vi "Main Read Data From VeriStand.vi"(8 "error in (no error)":errorcluster, 11 "J1939 Main Configuration":T1={"Parameters"={"J1939 XNET Settings"={"XNET Database"="", "XNET Cluster"="", "CAN Port"="", "Baud rate [Bd]"=0, "Termination"=0, "Incoming Rate"=0, "Outcoming Rate"=1, "Write Decimation"=1}, "Incoming Single Point Configuraiton"={"Incoming Single Point Frame"={"ID"=[], "Conversion"=[], "Channel Array Positions"=[], "Frame Length"=[]}, "Channel Pairs"={"Chan Refs"=[], "Previous Chan Values"=[]}, "Read FIFO"=refnum}, "Outgoing Cyclic Configuraiton"={"Outgoing Cyclic Frame"={"ID"=[], "Conversion"=[], "Channel Array Positions"=[], "Frame Length"=[], "Transmit Propreties"=[]}, "Channel Pairs"={"Block Data Refs"=[], "Previous Chan Values"=[]}, "Write FIFO"=refnum}, "J1939 Monitor Settings"={"J1939 Network Address"=0, "Name"=0}, "Simulated Addresses"=[], "Simulated Addresses LUT"=variant}, "Name"="", "J1939 Cluster"={"Processed Incoming"=refnum, "Current Device Address"=0, "Processed Outgoing"=refnum, "Process Outgoing"=refnum, "Name"=0}, "References"={"BAM Buffer"=refnum, "CM Buffer"=refnum, "CM Gen"=refnum, "BAM Gen"=refnum, "Address Claims"=refnum, "RQST"=refnum}, "StopRef"=refnum, "Frame In"="", "Frame Out"="", "Incoming Timeout"=0, "Outgoing Timeout"=0, "Listener ID"=refnum, "Parent VI Ref"=refnum, "Data Ref"=refnum, "Scale Ref"=refnum, "Incoming Direct Access"={"Offset"=0, "Length"=0}, "Outgoing Direct Access"={"Offset"=0, "Length"=0}, "vi reference"=refnum, "Name and Address"="", "Simulated Addresses"=[], "Simulated Addresses LUT"=variant} {"Simulated Addresses"."Simulated Addresses"."J1939 XNET Settings"."Name" format="%.0x"; "Simulated Addresses"."Simulated Addresses"."DM1 Data"."Data Reference" format="%.0x"; "Simulated Addresses"."Simulated Addresses"."DM1 Enable?"."Data Reference" format="%.0x"; "Simulated Addresses"."Simulated Addresses"."DM2 Data"."Data Reference" format="%.0x"; "Simulated Addresses"."Simulated Addresses"."DM2 Enable?"."Data Reference" format="%.0x"; "Parameters"."Simulated Addresses"."Simulated Addresses"."J1939 XNET Settings"."Name" format="%.0x"; "Parameters"."J1939 Monitor Settings"."Name" format="%.0x"; "Parameters"."Outgoing Cyclic Configuraiton"."Channel Pairs"."Block Data Refs"."Data Reference" format="%.0x"; "Parameters"."Outgoing Cyclic Configuraiton"."Outgoing Cyclic Frame"."Transmit Propreties"."Transmit Time" format="%#_p"; "Parameters"."J1939 XNET Settings"."Termination" items=["Off", "On"]; "Parameters"."Incoming Single Point Configuraiton"."Channel Pairs"."Chan Refs" format="%.0x"}) -> (0 "error out":errorcluster)   [LabVIEW 2013, in "J1939 Addon Engine.lvlib"]
uses:
  J1939 Addon Engine.lvlib
  Types/Configuration Cluster.ctl
  Types/Process Parameters.ctl
  Shared/Types/XNET Settings.ctl
  Types/Incoming Single Point Configuration.ctl
  Types/Incoming Single Point Frame Pairs.ctl
  Types/Incoming Single Point Channel Pairs.ctl
  <vilib>/NI Veristand/Custom Device API/Data Reference.ctl
  Types/Outgoing Cyclic Configuration.ctl
  Types/Outgoing Cyclic Frame Pairs.ctl
  Shared/Types/XNET Frame Event Properties.ctl
  Types/Outgoing Cyclic Channel Pairs.ctl
  <vilib>/NI Veristand/Custom Device API/Block Data Reference.ctl
  Shared/Types/Monitor Settings.ctl
  Types/Simulated Settings.ctl
  Shared/Types/Compiled Simulated Settings.ctl
  Types/DTC FIFOs.ctl
  Shared/J1939 Multi Packet Frame/Types/Setup Information Cluster.ctl
  <vilib>/xnet/xnet.llb/XNET Frame CAN.ctl
  <vilib>/xnet/xnet.llb/XNET Frame Type CAN.ctl
  Shared/J1939 Utilities/Types/CAN Outgoing Message Cluster.ctl
  Shared/J1939 Multi Packet Frame/Types/TP List References.ctl
  Shared/J1939 Multi Packet Frame/Types/BAM Buffer Connections List_Ref.ctl
  Shared/J1939 Multi Packet Frame/Types/Connection Mode Generation Connection Ref.ctl
  Shared/J1939 Multi Packet Frame/Types/BAM Generation Connections List_Ref.ctl
  Shared/J1939 Multi Packet Frame/Types/Address Table Reference.ctl
  Shared/J1939 Multi Packet Frame/Types/RQST Lookup Table Reference.ctl
  Stop FG/Stop Global Ref.ctl
  Diagnostics Addon/Source/Engine/SubVIs/Datatable Lookup DVR.ctl
  Shared/J1939 Multi Packet Frame/Types/RQST Comm Lookup Table_Ref.ctl
  Stop FG/Stop Global Commands.ctl
  Conversion Lookup Table Get Conversion Parameter.vi
  Data Lookup Table.vi
  Conversion Lookup Table.vi
  <vilib>/xnet/xnet.llb/XNET Convert.vi
  <vilib>/xnet/xnet.llb/XNET Convert (Signal to Frame Raw).vi
  Stop FG/Stop FG.lvlib
  Error Handling API/Error Handling API.lvlib
  Shared/J1939 Utilities/J1939 Utilities.lvlib
  <vilib>/NI Veristand/Custom Device API/Custom Device API.lvlib
  Shared/J1939 Addon Shared.lvlib
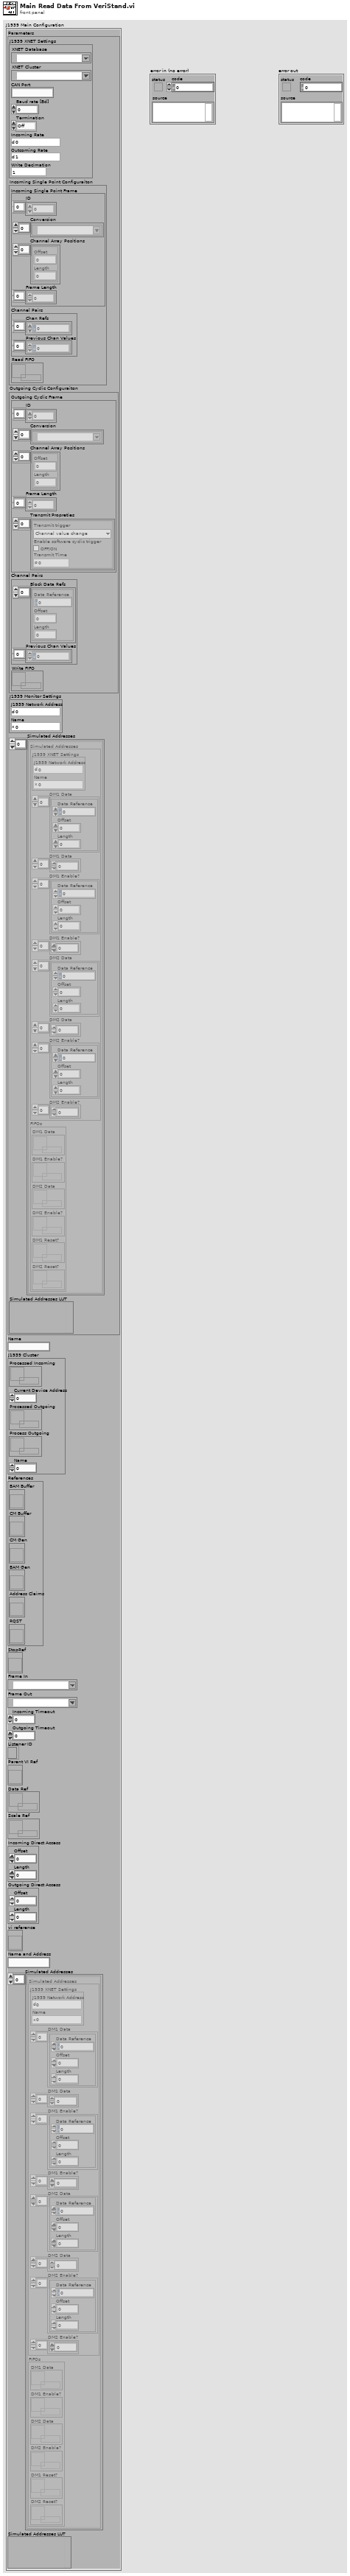
[diagram p1: front panel]
types:
  T1 = typedef "J1939 Addon Engine.lvlib/Configuration Cluster.ctl" = cluster{"Parameters":T2, "Name":string, "J1939 Cluster":T17, "References":T18, "StopRef":T24, "Frame In":refnum<k21>, "Frame Out":refnum<k21>, "Incoming Timeout":u32, "Outgoing Timeout":u32, "Listener ID":refnum<k5>, "Parent VI Ref":refnum<vi>, "Data Ref":refnum<data-value>, "Scale Ref":refnum<data-value>, "Incoming Direct Access":cluster{"Offset":u32, "Length":u32}, "Outgoing Direct Access":cluster{"Offset":u32, "Length":u32}, "vi reference":T25, "Name and Address":string, "Simulated Addresses":T14[], "Simulated Addresses LUT":variant}
  T2 = typedef "J1939 Addon Engine.lvlib/Process Parameters.ctl" = cluster{"J1939 XNET Settings":T3, "Incoming Single Point Configuraiton":T4, "Outgoing Cyclic Configuraiton":T8, "J1939 Monitor Settings":T13, "Simulated Addresses":T14[], "Simulated Addresses LUT":variant}
  T3 = typedef "J1939 Addon Shared.lvlib/XNET Settings.ctl" = cluster{"XNET Database":refnum<k21>, "XNET Cluster":refnum<k21>, "CAN Port":string, "Baud rate [Bd]":u32, "Termination":u32, "Incoming Rate":u32, "Outcoming Rate":u32, "Write Decimation":u32}
  T4 = typedef "J1939 Addon Engine.lvlib/Incoming Single Point Configuration.ctl" = cluster{"Incoming Single Point Frame":T5, "Channel Pairs":T6, "Read FIFO":refnum<k33>}
  T5 = typedef "J1939 Addon Engine.lvlib/Incoming Single Point Frame Pairs.ctl" = cluster{"ID":u32[], "Conversion":refnum<k21>[], "Channel Array Positions":cluster{"Offset":u32, "Length":u32}[], "Frame Length":u32[]}
  T6 = typedef "J1939 Addon Engine.lvlib/Incoming Single Point Channel Pairs.ctl" = cluster{"Chan Refs":T7[], "Previous Chan Values":dbl[]}
  T7 = typedef "Custom Device API.lvlib/Data Reference.ctl" = i32
  T8 = typedef "J1939 Addon Engine.lvlib/Outgoing Cyclic Configuration.ctl" = cluster{"Outgoing Cyclic Frame":T9, "Channel Pairs":T11, "Write FIFO":refnum<k33>}
  T9 = typedef "J1939 Addon Engine.lvlib/Outgoing Cyclic Frame Pairs.ctl" = cluster{"ID":u32[], "Conversion":refnum<k21>[], "Channel Array Positions":cluster{"Offset":u32, "Length":u32}[], "Frame Length":u32[], "Transmit Propreties":T10[]}
  T10 = typedef "J1939 Addon Shared.lvlib/XNET Frame Event Properties.ctl" = cluster{"Transmit trigger":enum16{"Channel value change"}, "Enable software cyclic trigger":bool, "Transmit Time":dbl}
  T11 = typedef "J1939 Addon Engine.lvlib/Outgoing Cyclic Channel Pairs.ctl" = cluster{"Block Data Refs":T12[], "Previous Chan Values":dbl[]}
  T12 = typedef "Custom Device API.lvlib/Block Data Reference.ctl" = cluster{"Data Reference":T7, "Offset":i32, "Length":i32}
  T13 = typedef "J1939 Addon Shared.lvlib/Monitor Settings.ctl" = cluster{"J1939 Network Address":u8, "Name":u64}
  T14 = typedef "J1939 Addon Engine.lvlib/Simulated Settings.ctl" = cluster{"Simulated Addresses":T15, "FIFOs":T16}
  T15 = typedef "J1939 Addon Shared.lvlib/Compiled Simulated Settings.ctl" = cluster{"J1939 XNET Settings":T13, "DM1 Data":T12[], "DM1 Data":dbl[], "DM1 Enable?":T12[], "DM1 Enable?":dbl[], "DM2 Data":T12[], "DM2 Data":dbl[], "DM2 Enable?":T12[], "DM2 Enable?":dbl[]}
  T16 = typedef "J1939 Addon Engine.lvlib/DTC FIFOs.ctl" = cluster{"DM1 Data":refnum<k33>, "DM1 Enable?":refnum<k33>, "DM2 Data":refnum<k33>, "DM2 Enable?":refnum<k33>, "DM1 Reset?":refnum<k33>, "DM2 Reset?":refnum<k33>}
  T17 = typedef "J1939 Addon Engine.lvlib/Setup Information Cluster.ctl" = cluster{"Processed Incoming":refnum<queue>, "Current Device Address":u8, "Processed Outgoing":refnum<queue>, "Process Outgoing":refnum<queue>, "Name":u64}
  T18 = typedef "J1939 Addon Engine.lvlib/TP List References.ctl" = cluster{"BAM Buffer":T19, "CM Buffer":T19, "CM Gen":T20, "BAM Gen":T21, "Address Claims":T22, "RQST":T23}
  T19 = typedef "J1939 Addon Engine.lvlib/BAM Buffer Connections List_Ref.ctl" = refnum<vi>
  T20 = typedef "J1939 Addon Engine.lvlib/Connection Mode Generation Connection Ref.ctl" = refnum<vi>
  T21 = typedef "J1939 Addon Engine.lvlib/BAM Generation Connections List_Ref.ctl" = refnum<vi>
  T22 = typedef "J1939 Addon Engine.lvlib/Address Table Reference.ctl" = refnum<vi>
  T23 = typedef "J1939 Addon Engine.lvlib/RQST Lookup Table Reference.ctl" = refnum<vi>
  T24 = typedef "J1939 Addon Engine.lvlib/Stop FG.lvlib/Stop Global Ref.ctl" = refnum<vi>
  T25 = typedef "J1939 Addon Engine.lvlib/RQST Comm Lookup Table_Ref.ctl" = refnum<vi>
  T26 = typedef "J1939 Addon Engine.lvlib/Stop FG.lvlib/Stop Global Commands.ctl" = enum16{"Write", "Read", "Reset"}
  T27 = typedef "J1939 Addon Shared.lvlib/J1939 Utilities.lvlib/CAN Outgoing Message Cluster.ctl" = cluster{"Identifier":u32, "Data":u8[]}
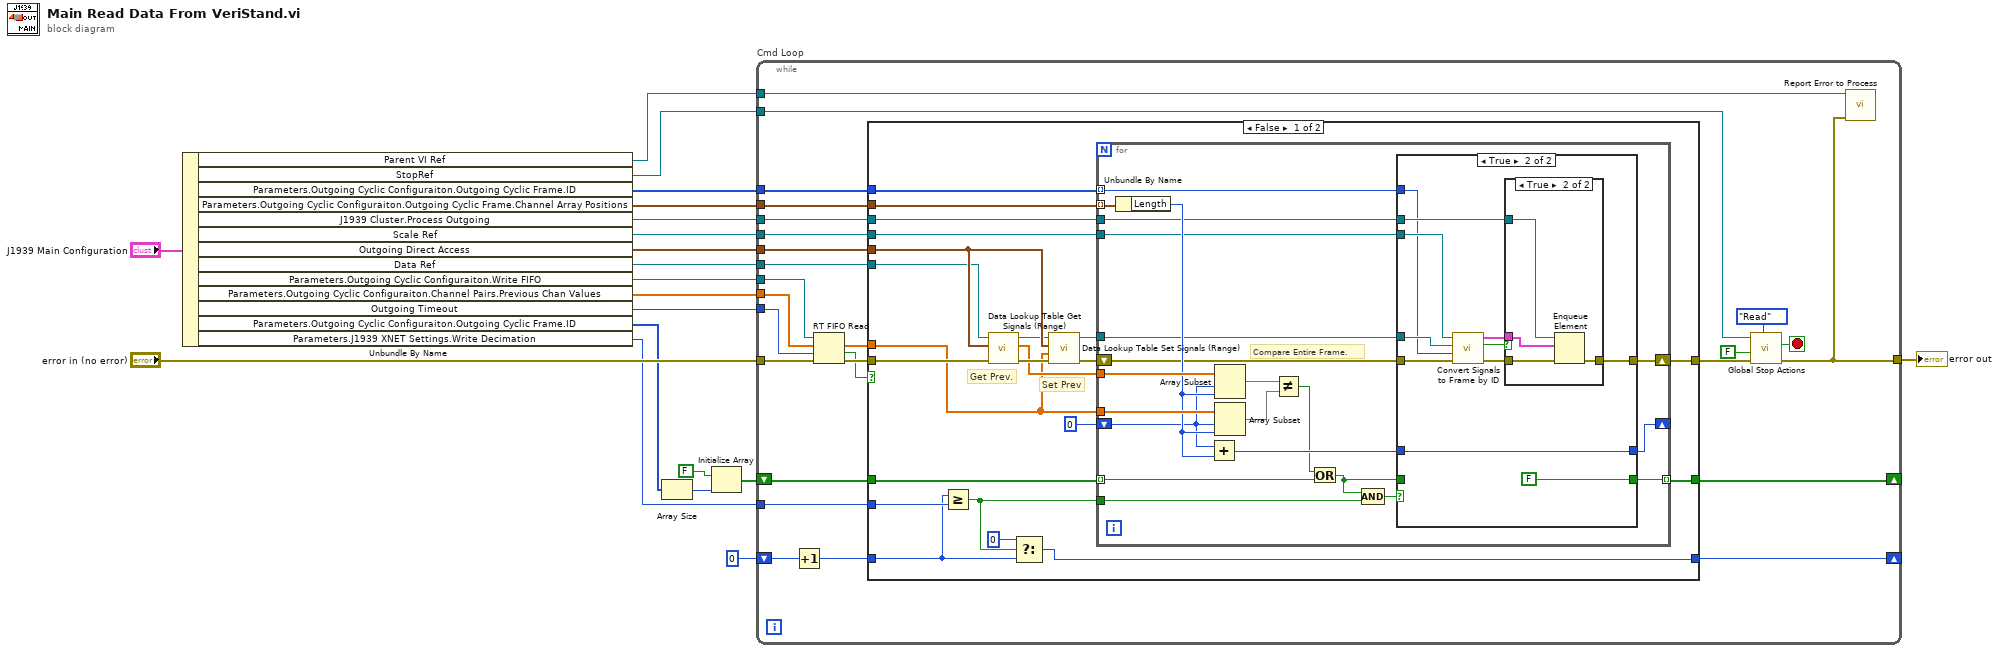
[diagram p0: block diagram]
diagram:
  n1 = Unbundle By Name("J1939 Main Configuration") -> ("Parent VI Ref"=w3:refnum<vi>, "StopRef"=w20:T24, "Parameters.Outgoing Cyclic Configuraiton.Outgoing Cyclic Frame.ID"=w14:u32[], "Parameters.Outgoing Cyclic Configuraiton.Outgoing Cyclic Frame.Channel Array Positions"=w2:cluster{"Offset":u32, "Length":u32}[], "J1939 Cluster.Process Outgoing"=w13:refnum<queue>, "Scale Ref"=w12:refnum<data-value>, "Outgoing Direct Access"=w11:cluster{"Offset":u32, "Length":u32}, "Data Ref"=w10:refnum<data-value>, "Parameters.Outgoing Cyclic Configuraiton.Write FIFO"=w8:refnum<k33>, "Parameters.Outgoing Cyclic Configuraiton.Channel Pairs.Previous Chan Values"=w9:dbl[], "Outgoing Timeout"=w7:u32, "Parameters.Outgoing Cyclic Configuraiton.Outgoing Cyclic Frame.ID"=w17:u32[], "Parameters.J1939 XNET Settings.Write Decimation"=w1:u32)
  n2 = Array Size(array=w17) -> (size(s)=w15:i32)
  n3 = Initialize Array(FALSE, w15) -> (w18:bool[])
  n4 = while "Cmd Loop" {
    tunnel: w13 -> [w37]
    tunnel: "error in (no error)" -> [w44]
    tunnel: [w33] -> w5
    tunnel: w8 -> [w43]
    tunnel: w11 -> [w40]
    tunnel: w10 -> [w39]
    tunnel: w14 -> [w42]
    tunnel: w12 -> [w35]
    tunnel: w9 -> [w34]
    shift-right: [w27] -> _
    shift-left: u32 0 -> [w29]
    shift-right: [w32] -> _
    shift-left: w18 -> [w31]
    tunnel: w1 -> [w30]
    tunnel: w20 -> [w25]
    tunnel: w7 -> [w23]
    tunnel: w3 -> [w22]
    tunnel: w2 -> [w21]
    stop <- w45 stop-if-true
    n5 = Increment(x=w29) -> (x+1=w28:u32)
    n6 = RT FIFO Read(0:w43, 1:w34, 2:w23, 3:w44) -> (9:w38:dbl[], 10:w24:bool, 11:w41:errorcluster)  [unwired: 2 out]
    n7 = case shown="False" w24 {
      tunnel: w42 -> [w48 _]
      tunnel: w41 -> [w66 w111]
      tunnel: w40 -> [w64 _]
      tunnel: w39 -> [w63 _]
      tunnel: w38 -> [w60 _]
      tunnel: w37 -> [w49 _]
      tunnel: [w58 w111] -> w36
      tunnel: w35 -> [w57 _]
      tunnel: [w56 w110] -> w32
      tunnel: w31 -> [w55 w110]
      tunnel: w30 -> [w54 _]
      tunnel: w28 -> [w52 w109]
      tunnel: [w50 w109] -> w27
      tunnel: w21 -> [w47 _]
      frame False {
        # "Set Prev"
        # "Get Prev."
        n8 = Greater Or Equal?(x=w52, y=w54) -> (x >= y?=w53:bool)
        n9 = call "Data Lookup Table Get Signals (Range).vi"("error in (no error)"=w66, "Direct Access"=w64, "Data Ref"=w63) -> ("error out"=w65:errorcluster, "Signals"=w61:dbl[], "Data Ref out"=w62:refnum<data-value>)  [unwired: 6 in]
        n10 = Select(t=0, s=w53, f=w52) -> (s? t:f=w50:u32)
        n11 = call "Data Lookup Table Set Signals (Range).vi"("error in (no error)"=w65, "Signals"=w60, "Direct Access"=w64, "Data Ref"=w62) -> ("error out"=w68:errorcluster, "Data Ref out"=w67:refnum<data-value>)  [unwired: 6 in]
        n12 = for {
          tunnel: w47 -> [w89] mode=indexing
          tunnel: w67 -> [w80]
          tunnel: w61 -> [w88]
          tunnel: w60 -> [w87]
          shift-right: [w74] -> _
          shift-left: u32 0 -> [w85]
          shift-right: [w83] -> w58
          shift-left: w68 -> [w84]
          tunnel: w49 -> [w82]
          tunnel: w48 -> [w81] mode=indexing
          tunnel: w57 -> [w79]
          tunnel: [w78] -> w56 mode=indexing
          tunnel: w55 -> [w73] mode=indexing
          tunnel: w53 -> [w76]
          # "Compare Entire Frame."
          n13 = Unbundle By Name(w89) -> ("Length"=w86:u32)
          n14 = Add(x=w85, y=w86) -> (x+y=w75:u32)
          n15 = Array Subset(array=w88, index=w85, length=w86) -> (w69:dbl[])
          n16 = Array Subset(array=w87, index=w85, length=w86) -> (w70:dbl[])
          n17 = Not Equal?(x=w69, y=w70) -> (x != y?=w72:bool)
          n18 = Or(x=w72, y=w73) -> (x .or. y?=w71:bool)
          n19 = Compound Arithmetic op=AND(w71, w76) -> (w77:bool)
          n20 = case shown="True" w77 {
            tunnel: w84 -> [w92 w101]
            tunnel: [w92 w103] -> w83
            tunnel: w82 -> [_ w102]
            tunnel: w81 -> [_ w94]
            tunnel: w80 -> [_ w98]
            tunnel: w79 -> [_ w97]
            tunnel: [w90 FALSE] -> w78
            tunnel: w75 -> [w91 w95]
            tunnel: [w91 w95] -> w74
            tunnel: w71 -> [w90 _]
            frame False {
            }
            frame True {
              n21 = call "Convert Signals to Frame by ID.vi"("error in (no error)"=w101, "ID"=w94, "Data Ref"=w98, "Scale Ref"=w97) -> ("error out"=w100:errorcluster, "Found?"=w93:bool, "Frame"=w99:T27)  [unwired: 5 in]
              n22 = case shown="True" w93 {
                tunnel: [w104 w108] -> w103
                tunnel: w102 -> [_ w107]
                tunnel: w100 -> [w104 w106]
                tunnel: w99 -> [_ w105]
                frame False {
                }
                frame True {
                  n23 = Enqueue Element(queue=w107, element=w105, error in (no error)=w106) -> (error out=w108:errorcluster)  [unwired: 3 out]
                }
              }
            }
          }
        }
      }
      frame True {
      }
    }
    n24 = call "Global Stop Actions.vi"("Command"=Stop_Global_Commands."Read", "error in (no error)"=w36, "Stop on Error?"=FALSE, "vi reference"=w25) -> ("error out"=w33:errorcluster, "Latched Stop"=w45:bool)  [unwired: 5 in, 1 out]
    n25 = call "Report Error to Process.vi"("Error"=w33, "This VI"=w22) -> ()  [unwired: 10 in]
  }
  "error out" <- w5
